vi "Loop unroll - nested.vi"(1 "Script":string="filename\nloop(3){pump /1Q #query pump\npump /1? #report absolute plunger position\npump /1?6 #report valve position}\nloop(2){pump /2Q #query pump}") -> (0 "Output":string)   [LabVIEW 2019]
panel:
  # "Examples\n\nfilename\nloop(3){pump /1Q #query pump\npump /1? #report absolute plunger position\npump /1?6 #report valve position}\nloop(2){pump /2Q #query pump}\n\nfilename\nloop(3){pump /1Q #query pump\npump /1? #report absolute plunger position\npump /1?6 #report valve position\nloop(2){pump /2Q #query pump}}\n\nstuff\nloop(3){repeat1\nloop(2){repeat2}}\n\nfilename\nloop(3){pump /1Q #query pump\npump /1? #report absolute plunger position\npump /1?6 #report valve position\npump /2Q #query pump\npump /2Q #query pump}"
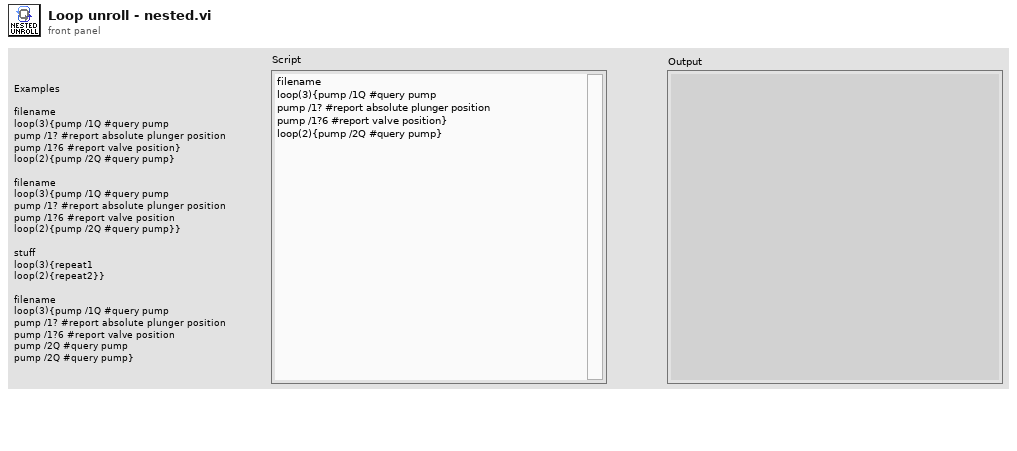
[diagram p1: front panel]
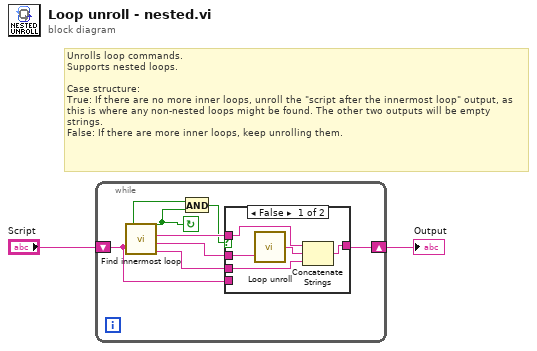
[diagram p0: block diagram]
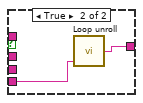
[diagram p2: hidden frame]
diagram:
  # "Unrolls loop commands.\nSupports nested loops.\n\nCase structure:\nTrue: If there are no more inner loops, unroll the \"script after the innermost loop\" output, as this is where any non-nested loops might be found. The other two outputs will be empty strings.\nFalse: If there are more inner loops, keep unrolling them."
  n1 = while {
    shift-right: [w9] -> w1
    shift-left: "Script" -> [w10]
    stop <- w3 continue-if-true
    n2 = call "Find innermost loop.vi"("Script"=w10) -> ("No nested loops?"=w4:bool, "Any more loops?"=w3:bool, "Script before innermost loop"=w6:string, "Innermost loop"=w8:string, "Script after innermost loop"=w7:string)  [unwired: 2 out]
    n3 = And(x=w4, y=w3) -> (x .and. y?=w5:bool)
    n4 = case shown="False" w5 {
      tunnel: [w14 w17] -> w9
      tunnel: w8 -> [w15 _]
      tunnel: w7 -> [w11 _]
      tunnel: w6 -> [w13 _]
      tunnel: w10 -> [_ w16]
      frame False {
        n5 = call "Loop unroll.vi"("Loop"=w15) -> ("Unrolled loop"=w12:string)  [unwired: 2 in]
        n6 = Concatenate Strings(w13, w12, w11) -> (w14:string)
      }
      frame True {
        n7 = call "Loop unroll.vi"("Loop"=w16) -> ("Unrolled loop"=w17:string)  [unwired: 2 in]
      }
    }
  }
  "Output" <- w1
